vi "stations save Station.vi"(8 "error in (no error)":errorcluster, 9 "Post Data (empty)":T3, 10 "Station ID (\"\")":string, 11 "Connection Refnum":T2) -> (0 "error out":errorcluster, 2 "Station Record":T1, 3 "dup Connection Refnum":T2)   [LabVIEW 2011]
uses:
  Addons/internet/utils/keyedarr.llb/Keyed Array.ctl
  SI.LIB/ODBC/SQL Controls/Connection Refnum.ctl
  server/database/Stations/Station Record.ctl
  Addons/internet/utils/strutil.llb/Case Matching.ctl
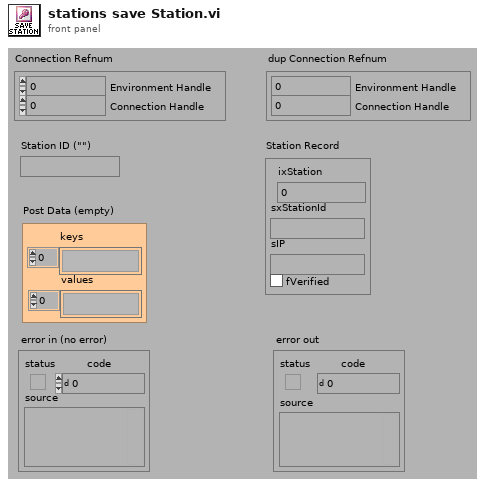
[diagram p1: front panel]
types:
  T1 = typedef "Station Record.ctl" = cluster{"ixStation":i32, "sxStationId":string, "sIP":string, "fVerified":bool}
  T2 = typedef "Connection Refnum.ctl" = cluster{"Environment Handle":i32, "Connection Handle":i32}
  T3 = typedef "Keyed Array.ctl" = cluster{"keys":string[], "values":string[]}
  T4 = typedef "Case Matching.ctl" = enum16{"a != A", "a == A", "system"}
  T5 = typedef "Instrument Record.ctl" = cluster{"ixInstrument":i32, "sxInstrumentId":string, "sDriverId":string, "sDriverType":string, "sSerialNumber":string, "tLastCalibration":timestamp, "tCalibrationDue":timestamp, "sConfiguration":string}
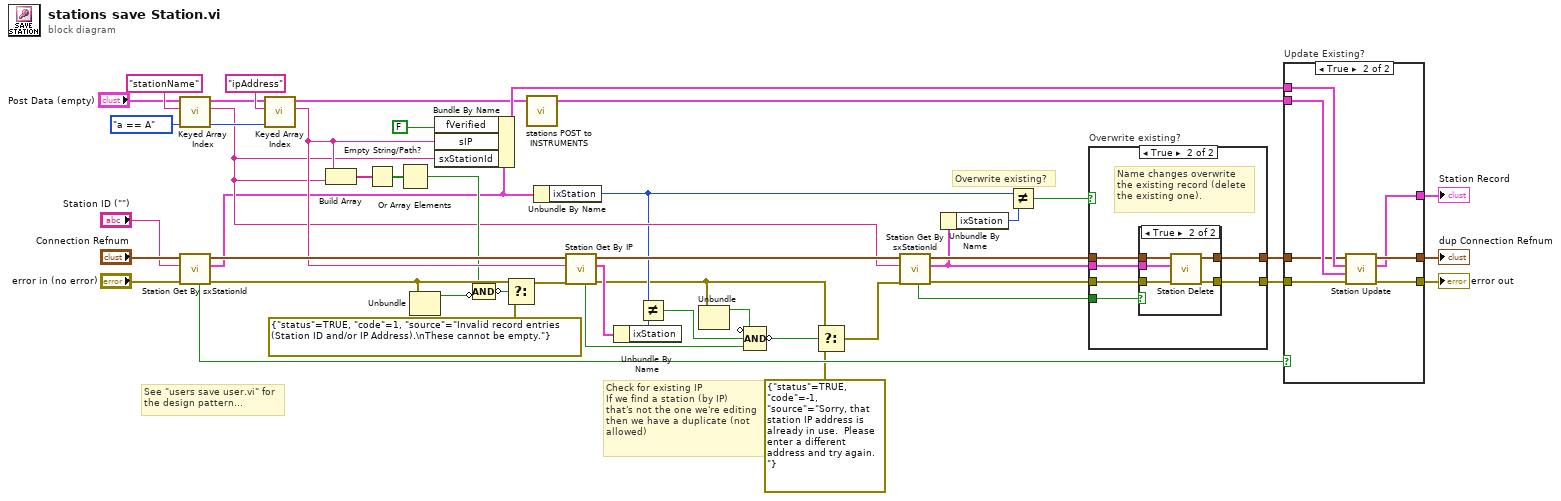
[diagram p0: block diagram]
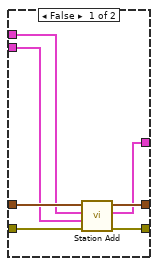
[diagram p4: hidden frame]
diagram:
  w29 = Case_Matching."a == A" ("case matching (sensitive)")
  # "Overwrite existing?"
  # "See \"users save user.vi\" for\nthe design pattern..."
  # "Check for existing IP\nIf we find a station (by IP)\nthat's not the one we're editing\nthen we have a duplicate (not\nallowed)"
  n1 = call "Keyed Array Index.vi"("case matching (sensitive)"=w29, "key"="stationName", "array in"="Post Data (empty)") -> ("value"=w16:string, "duplicate array"=w30:T3)  [unwired: 1 in, 2 out]
  n2 = call "Station Get By sxStationId.vi"("error in (no error)"="error in (no error)", "sxStationId (\"\")"="Station ID (\"\")", "Connection Refnum"="Connection Refnum") -> ("error out"=w22:errorcluster, "Station Record"=w14:T1, "Connection Refnum"=w38:T2, "Data Present?"=w28:bool)  [unwired: 5 out]
  n3 = call "Keyed Array Index.vi"("case matching (sensitive)"=w29, "key"="ipAddress", "array in"=w30) -> ("value"=w27:string, "duplicate array"=w44:T3)  [unwired: 1 in, 2 out]
  n4 = Build Array(w27, w16) -> (w26:string[])
  n5 = Empty String/Path?(string/path=w26) -> (empty?=w25:bool[])
  n6 = Or Array Elements(Boolean array=w25) -> (logical OR=w19:bool)
  n7 = Unbundle(w22) -> ("status"=w20:bool)  [unwired: 2 out]
  n8 = Bundle By Name(cluster=w14, "fVerified"=FALSE, "sIP"=w27, "sxStationId"=w16) -> (w46:T1)
  n9 = Compound Arithmetic op=AND(w19, invert w20) -> (invert w24:bool)
  n10 = Select(t=w22, s=w24, f=errorcluster {"status"=TRUE, "code"=1, "source"="Invalid record entries (Station ID and/or IP Address).\nThese cannot be empty."} ("t")) -> (s? t:f=w23:errorcluster)
  n11 = call "stations POST to INSTRUMENTS.vi"("POST (empty)"=w44) -> ("INSTRUMENTS on Station"=w41:T5[])  [unwired: 4 out]
  n12 = Unbundle By Name(w14) -> ("ixStation"=w15:i32)
  n13 = call "Station Get By IP.vi"("error in (no error)"=w23, "IP or Name (\"\")"=w27, "Connection Refnum"=w38) -> ("error out"=w3:errorcluster, "Station Record"=w37:T1, "Connection Refnum"=w17:T2, "Data Present?"=w35:bool)  [unwired: 5 out]
  n14 = Unbundle By Name(w37) -> ("ixStation"=w36:i32)
  n15 = Not Equal?(x=w15, y=w36) -> (x != y?=w34:bool)
  n16 = Unbundle(w3) -> ("status"=w4:bool)  [unwired: 2 out]
  n17 = Compound Arithmetic op=AND(invert w4, w34, w35) -> (invert w1:bool)
  n18 = Select(t=w3, s=w1, f=errorcluster {"status"=TRUE, "code"=-1, "source"="Sorry, that station IP address is already in use.  Please enter a different address and try again."} ("error out")) -> (s? t:f=w2:errorcluster)
  n19 = call "Station Get By sxStationId.vi"("error in (no error)"=w2, "sxStationId (\"\")"=w16, "Connection Refnum"=w17) -> ("error out"=w11:errorcluster, "Station Record"=w8:T1, "Connection Refnum"=w12:T2, "Data Present?"=w6:bool)  [unwired: 5 out]
  n20 = Unbundle By Name(w8) -> ("ixStation"=w13:i32)
  n21 = Not Equal?(x=w15, y=w13) -> (x != y?=w7:bool)
  n22 = case "Overwrite existing?" shown="True" w7 {
    tunnel: w11 -> [w48 w51]
    tunnel: w12 -> [w49 w53]
    tunnel: [w48 w55] -> w9
    tunnel: [w49 w54] -> w10
    tunnel: w8 -> [_ w52]
    tunnel: w6 -> [_ w50]
    frame False {
    }
    frame True {
      # "Name changes overwrite\nthe existing record (delete\nthe existing one)."
      n23 = case shown="True" w50 {
        tunnel: w51 -> [w56 w62]
        tunnel: [w56 w61] -> w55
        tunnel: w53 -> [w57 w60]
        tunnel: [w57 w59] -> w54
        tunnel: w52 -> [_ w58]
        frame False {
        }
        frame True {
          n24 = call "Station Delete.vi"("error in (no error)"=w62, "TestStation Record"=w58, "Connection Refnum"=w60) -> ("error out"=w61:errorcluster, "Connection Refnum"=w59:T2)  [unwired: 7 out]
        }
      }
    }
  }
  n25 = case "Update Existing?" shown="True" w28 {
    tunnel: w10 -> [w69 w71]
    tunnel: w9 -> [w68 w70]
    tunnel: w46 -> [w67 w76]
    tunnel: [w65 w75] -> w42
    tunnel: [w66 w74] -> w43
    tunnel: w41 -> [w64 w73]
    tunnel: [w63 w72] -> w18
    frame False {
      n26 = call "Station Add.vi"("error in (no error)"=w68, "Instruments on Station (none)"=w64, "Station Record (empty)"=w67, "Connection Refnum"=w69) -> ("error out"=w65:errorcluster, "New Station Record"=w63:T1, "Connection Refnum"=w66:T2)  [unwired: 5 out]
    }
    frame True {
      n27 = call "Station Update.vi"("error in (no error)"=w70, "Instruments (none)"=w73, "Station Record (empty)"=w76, "Connection Refnum"=w71) -> ("error out"=w75:errorcluster, "Station"=w72:T1, "Connection Refnum"=w74:T2)  [unwired: 5 out]
    }
  }
  "error out" <- w42
  "dup Connection Refnum" <- w43
  "Station Record" <- w18
